vi "Obtain Data Notifier.vi"(8 "error in (no error)":errorcluster, 10 "Create New?":bool) -> (0 "error out":errorcluster, 2 "Data Notifiers":T1)   [LabVIEW 2015, in "Tool Module.lvlib"]
uses:
  Tool Module.lvlib
  _Data Notifiers Cluster--typedef.ctl
  _Sample Data Rtn Cluster--typedef.ctl
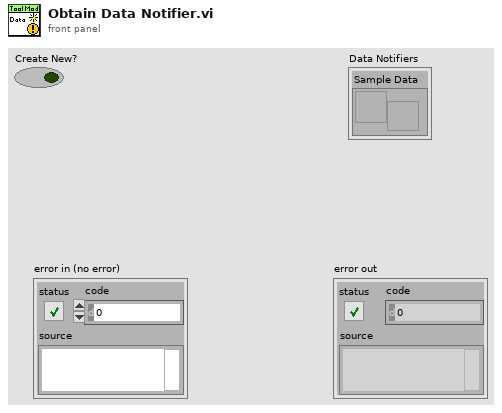
[diagram p1: front panel]
types:
  T1 = typedef "Tool Module.lvlib/_Data Notifiers Cluster--typedef.ctl" = cluster{"Sample Data":refnum<notifier>}
  T2 = typedef "Tool Module.lvlib/_Sample Data Rtn Cluster--typedef.ctl" = cluster{"Inspecting":bool, "Scan Data Array":u32[]}
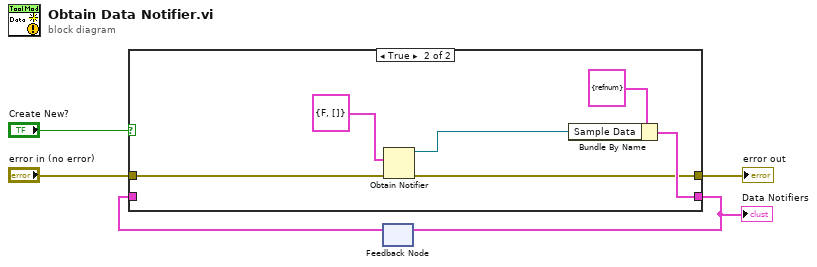
[diagram p0: block diagram]
diagram:
  n1 = feedback #1() -> (w1:T1)  [unwired: 1 in]
  n2 = case shown="True" "Create New?" {
    tunnel: [w7 w10] -> w2
    tunnel: "error in (no error)" -> [w6 w9]
    tunnel: [w6 w8] -> w3
    tunnel: w1 -> [w7 _]
    frame False {
    }
    frame True {
      n3 = Obtain Notifier(notification data type=T2 {"Inspecting"=FALSE, "Scan Data Array"=[]} ("_Full Scan Data Rtn Cluster"), error in (no error)=w9) -> (notifier out=w12:refnum<notifier>, error out=w8:errorcluster)  [unwired: 2 in, 1 out]
      n4 = Bundle By Name(cluster=T1 {"Sample Data"=refnum} ("_Data Notifiers Cluster--typedef"), "Sample Data"=w12) -> (w10:T1)
    }
  }
  "error out" <- w3
  "Data Notifiers" <- w2
  n5 = feedback-in #1(w2) -> ()
